vi "PicowattAVS47Monitor.vi"() -> ()   [LabVIEW 2018]
uses:
  Utility/Monitor Communication/PicowattAVS47/PicowattAVS47-Cluster.ctl
  Instrument_Setup.vi
  Global/Global Variables/Data_Display_global.vi
panel:
  in  "?":bool
  out "Picowatt AVS47/TS530 Cluster":T1 {"AVS Excitation" items=["no Exc", "3uV", "10uV", "30uV", "100uV", "300uV", "1mV", "3mV"]}
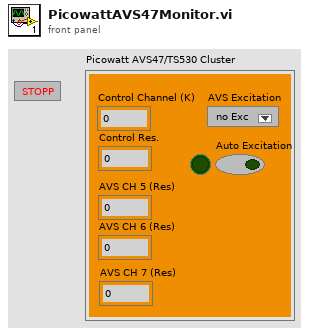
[diagram p1: front panel]
types:
  T1 = typedef "PicowattAVS47-Cluster.ctl" = cluster{"Control Channel (K)":dbl, "AVS CH 5 (Res)":dbl, "AVS CH 6 (Res) ":dbl, "AVS CH 7 (Res) ":dbl, "Control Res.":dbl, "Auto Excitation":bool, "Auto activatet":bool, "AVS Excitation":i16}
  T2 = typedef "AVS-Control-Cluster.ctl" = cluster{"AVS Excitation":i16, "Auto Excitation":bool}
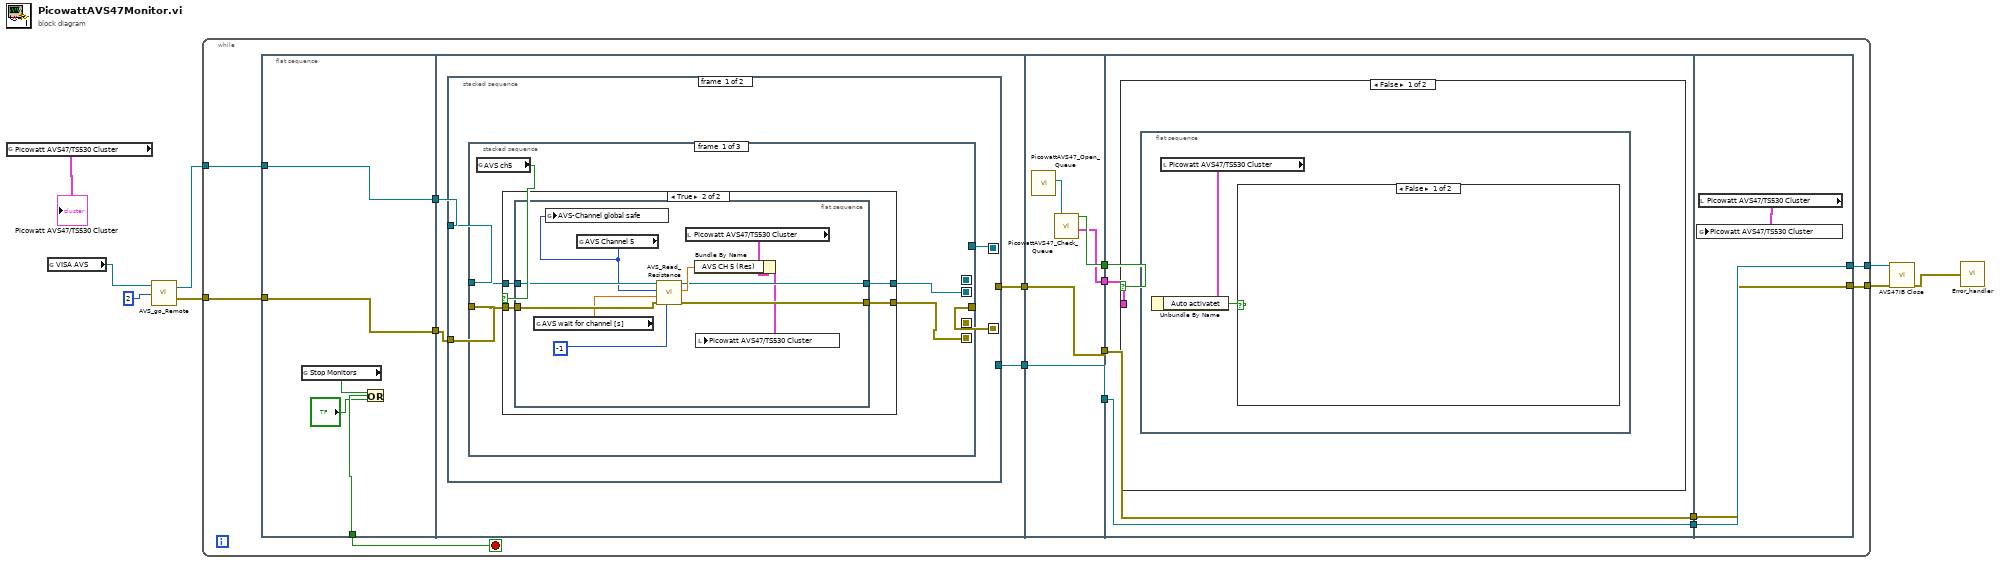
[diagram p0: block diagram]
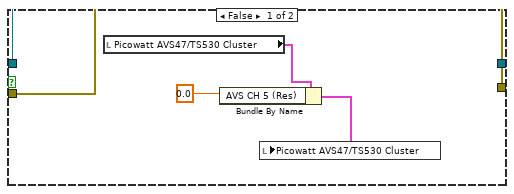
[diagram p2: hidden frame]
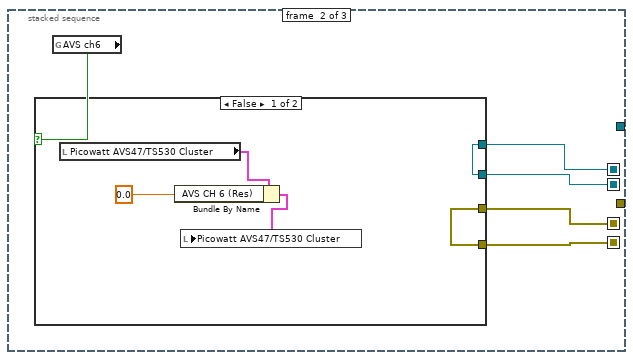
[diagram p3: hidden frame]
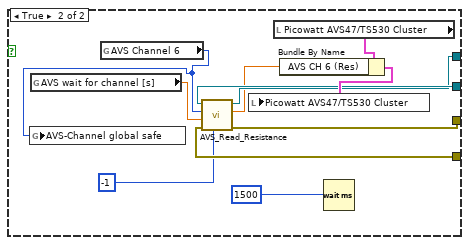
[diagram p4: hidden frame]
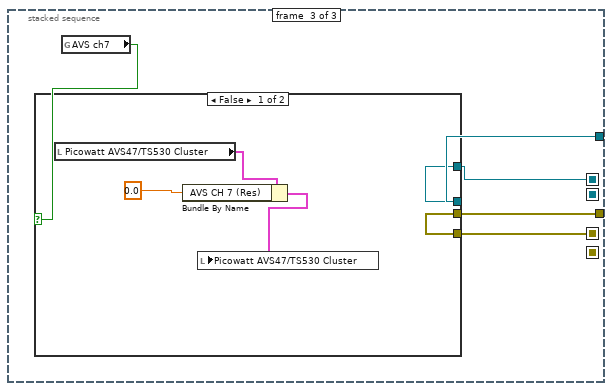
[diagram p5: hidden frame]
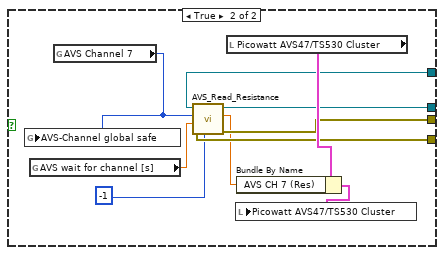
[diagram p6: hidden frame]
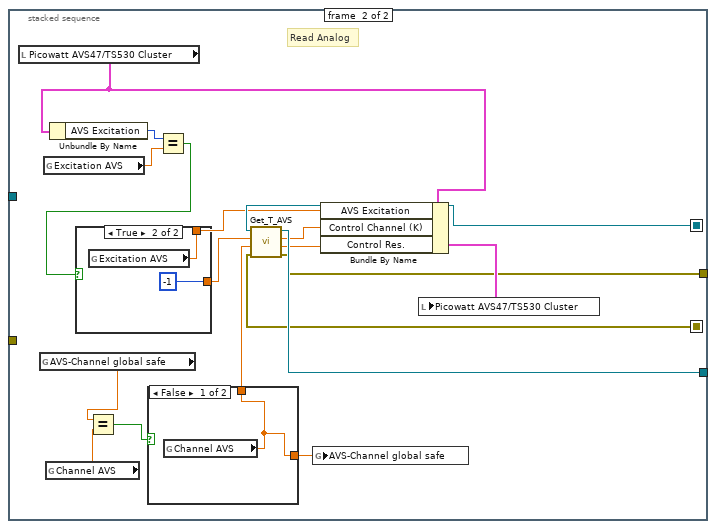
[diagram p7: hidden frame]
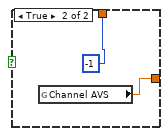
[diagram p8: hidden frame]
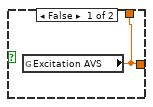
[diagram p9: hidden frame]
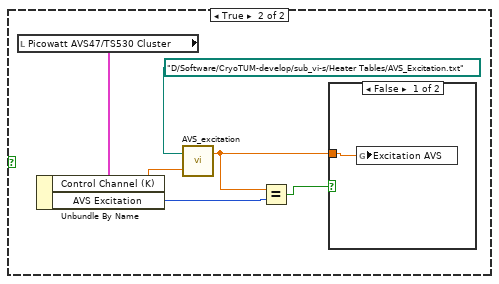
[diagram p10: hidden frame]
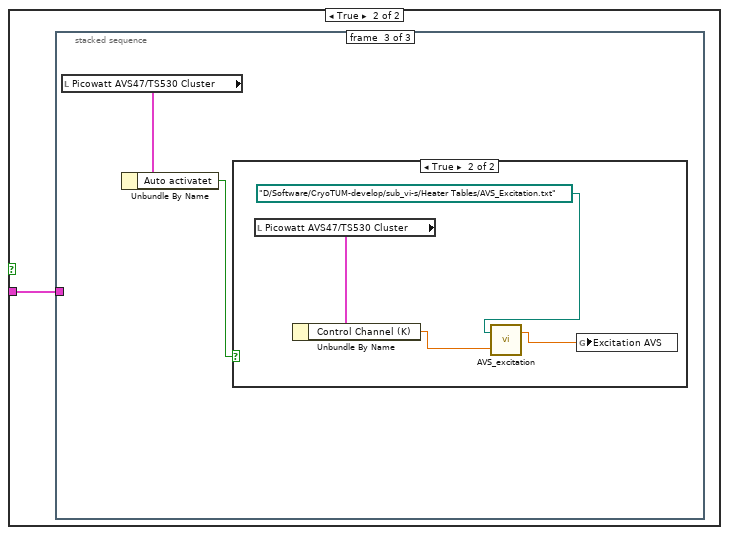
[diagram p12: hidden frame]
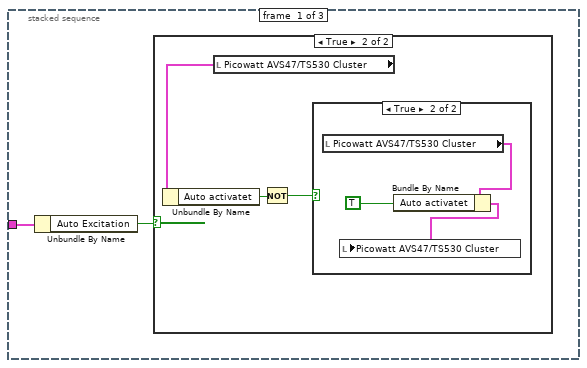
[diagram p13: hidden frame]
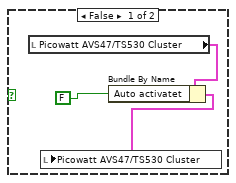
[diagram p15: hidden frame]
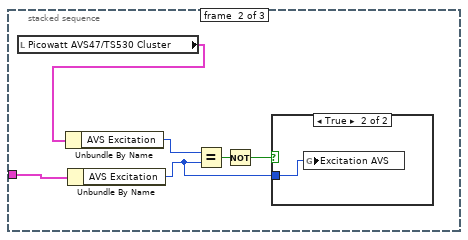
[diagram p16: hidden frame]
diagram:
  n1 = global read "Data_Display_global.vi" "Picowatt AVS47/TS530 Cluster"() -> (→"Picowatt AVS47/TS530 Cluster":T1)
  n2 = global read "Instrument_Setup.vi" "VISA AVS"() -> (w7:refnum<visa-resource-name>)
  n3 = call "AVS_go_Remote.vi"("Timeout (sec)"=i16 2, "VISA-AVS"=w7) -> ("error out"=w8:errorcluster, "dup VISA session"=w6:refnum<visa-resource-name>)  [unwired: 1 in]
  n4 = while {
    tunnel: w8 -> [w18]
    tunnel: w6 -> [w17]
    tunnel: [w10] -> w3
    tunnel: [w9] -> w2
    stop <- w23 stop-if-true
    n5 = flat-sequence {
      tunnel: [w28] -> w23
      tunnel: [w24] -> w22
      tunnel: [w25] -> w19
      tunnel: w18 -> [w25]
      tunnel: w17 -> [w24]
      tunnel: w22 -> [w32]
      tunnel: w19 -> [w31]
      tunnel: [w30] -> w16
      tunnel: [w29] -> w15
      tunnel: [w129] -> w21
      tunnel: [w128] -> w20
      tunnel: w16 -> [w126]
      tunnel: w15 -> [w127]
      tunnel: [w127] -> w14
      tunnel: [w126] -> w13
      tunnel: w21 -> [w134]
      tunnel: w20 -> [w133]
      tunnel: w14 -> [w131]
      tunnel: w13 -> [w132]
      tunnel: [w132] -> w12
      tunnel: [w131] -> w11
      tunnel: w12 -> [w170]
      tunnel: w11 -> [w169]
      tunnel: [w170] -> w10
      tunnel: [w169] -> w9
      frame #0 {
        n6 = global read "Data_Display_global.vi" "Stop Monitors"() -> (w26:bool)
        n7 = Or(x=w26, y="?") -> (x .or. y?=w28:bool)
      }
      frame #1 {
        n8 = stacked-sequence {
          seq-local: [w34 _] -> [_ w118]
          seq-local: [w33 _] -> [_ w116]
          tunnel: w32 -> [w35 _]
          tunnel: w31 -> [w36 _]
          tunnel: [_ w117] -> w30
          tunnel: [_ w115] -> w29
          frame #0 {
            n9 = stacked-sequence {
              seq-local: [w40 _ _] -> [_ w64 _]
              seq-local: [_ w63 _] -> [_ _ w85]
              seq-local: [w37 _ _] -> [_ w62 _]
              seq-local: [_ w61 _] -> [_ _ w83]
              tunnel: w36 -> [w39 _ _]
              tunnel: [_ _ w84] -> w33
              tunnel: w35 -> [w38 _ _]
              tunnel: [_ _ w82] -> w34
              frame #0 {
                n10 = global read "Instrument_Setup.vi" "AVS ch5"() -> (w41:bool)
                n11 = case shown="True" w41 {
                  tunnel: [w46 w50] -> w40
                  tunnel: w39 -> [w46 w49]
                  tunnel: w38 -> [w45 w48]
                  tunnel: [w45 w47] -> w37
                  frame False {
                    n12 = local read "Picowatt AVS47/TS530 Cluster"() -> (w44:T1)
                    n13 = Bundle By Name(cluster=w44, "AVS CH 5 (Res)"=0.0) -> (w42:T1)
                    n14 = local write "Picowatt AVS47/TS530 Cluster"(w42) -> ()
                  }
                  frame True {
                    n15 = flat-sequence {
                      tunnel: w49 -> [w58]
                      tunnel: w48 -> [w57]
                      tunnel: [w59] -> w50
                      tunnel: [w54] -> w47
                      frame #0 {
                        n16 = global read "Instrument_Setup.vi" "AVS wait for channel [s]"() -> (w56:dbl)
                        n17 = global read "Instrument_Setup.vi" "AVS Channel 5"() -> (w52:enum16{"1", "2", "3", "4", "5", "6", "7"})
                        n18 = global write "Data_Display_global.vi" "AVS-Channel global safe"(w52) -> ()
                        n19 = call "AVS_Read_Resistance.vi"("AVS-Excitation"=i8 -1, "error in (no error)"=w58, "Wait for channel (s)"=w56, "AVS Channel"=w52, "AVS-VISA"=w57) -> ("error out"=w59:errorcluster, "AVS Resistance reading"=w55:dbl, "dup AVS-VISA"=w54:refnum<visa-resource-name>)  [unwired: 2 in]
                        n20 = local read "Picowatt AVS47/TS530 Cluster"() -> (w60:T1)
                        n21 = Bundle By Name(cluster=w60, "AVS CH 5 (Res)"=w55) -> (w51:T1)
                        n22 = local write "Picowatt AVS47/TS530 Cluster"(w51) -> ()
                      }
                    }
                  }
                }
              }
              frame #1 {
                n23 = global read "Instrument_Setup.vi" "AVS ch6"() -> (w65:bool)
                n24 = case shown="False" w65 {
                  tunnel: w64 -> [w70 w79]
                  tunnel: [w70 w78] -> w63
                  tunnel: w62 -> [w69 w77]
                  tunnel: [w69 w76] -> w61
                  frame False {
                    n25 = local read "Picowatt AVS47/TS530 Cluster"() -> (w68:T1)
                    n26 = Bundle By Name(cluster=w68, "AVS CH 6 (Res)"=0.0) -> (w66:T1)
                    n27 = local write "Picowatt AVS47/TS530 Cluster"(w66) -> ()
                  }
                  frame True {
                    n28 = global read "Instrument_Setup.vi" "AVS wait for channel [s]"() -> (w75:dbl)
                    n29 = global read "Instrument_Setup.vi" "AVS Channel 6"() -> (w72:enum16{"1", "2", "3", "4", "5", "6", "7"})
                    n30 = global write "Data_Display_global.vi" "AVS-Channel global safe"(w72) -> ()
                    n31 = call "AVS_Read_Resistance.vi"("AVS-Excitation"=i8 -1, "error in (no error)"=w79, "Wait for channel (s)"=w75, "AVS Channel"=w72, "AVS-VISA"=w77) -> ("error out"=w78:errorcluster, "AVS Resistance reading"=w74:dbl, "dup AVS-VISA"=w76:refnum<visa-resource-name>)  [unwired: 2 in]
                    n32 = local read "Picowatt AVS47/TS530 Cluster"() -> (w81:T1)
                    n33 = Bundle By Name(cluster=w81, "AVS CH 6 (Res)"=w74) -> (w80:T1)
                    n34 = local write "Picowatt AVS47/TS530 Cluster"(w80) -> ()
                    n35 = Wait (ms)(milliseconds to wait=1500) -> ()  [unwired: 1 out]
                  }
                }
              }
              frame #2 {
                n36 = global read "Instrument_Setup.vi" "AVS ch7"() -> (w86:bool)
                n37 = case shown="False" w86 {
                  tunnel: w85 -> [w91 w100]
                  tunnel: [w91 w99] -> w84
                  tunnel: w83 -> [w90 w98]
                  tunnel: [w90 w97] -> w82
                  frame False {
                    n38 = local read "Picowatt AVS47/TS530 Cluster"() -> (w89:T1)
                    n39 = Bundle By Name(cluster=w89, "AVS CH 7 (Res)"=0.0) -> (w87:T1)
                    n40 = local write "Picowatt AVS47/TS530 Cluster"(w87) -> ()
                  }
                  frame True {
                    n41 = global read "Instrument_Setup.vi" "AVS wait for channel [s]"() -> (w96:dbl)
                    n42 = global read "Instrument_Setup.vi" "AVS Channel 7"() -> (w93:enum16{"1", "2", "3", "4", "5", "6", "7"})
                    n43 = global write "Data_Display_global.vi" "AVS-Channel global safe"(w93) -> ()
                    n44 = call "AVS_Read_Resistance.vi"("AVS-Excitation"=i8 -1, "error in (no error)"=w100, "Wait for channel (s)"=w96, "AVS Channel"=w93, "AVS-VISA"=w98) -> ("error out"=w99:errorcluster, "AVS Resistance reading"=w95:dbl, "dup AVS-VISA"=w97:refnum<visa-resource-name>)  [unwired: 2 in]
                    n45 = local read "Picowatt AVS47/TS530 Cluster"() -> (w101:T1)
                    n46 = Bundle By Name(cluster=w101, "AVS CH 7 (Res)"=w95) -> (w92:T1)
                    n47 = local write "Picowatt AVS47/TS530 Cluster"(w92) -> ()
                  }
                }
              }
            }
          }
          frame #1 {
            # "Read Analog"
            n48 = local read "Picowatt AVS47/TS530 Cluster"() -> (w102:T1)
            n49 = global read "Data_Display_global.vi" "AVS-Channel global safe"() -> (w108:dbl)
            n50 = global read "Instrument_Setup.vi" "Excitation AVS"() -> (w111:dbl)
            n51 = global read "Instrument_Setup.vi" "Channel AVS"() -> (w107:dbl)
            n52 = Unbundle By Name(w102) -> ("AVS Excitation"=w112:i16)
            n53 = Equal?(x=w108, y=w107) -> (x = y?=w106:bool)
            n54 = case shown="False" w106 {
              tunnel: [w120 -1] -> w105
              tunnel: [w120 w121] -> w104
              frame False {
                n55 = global read "Instrument_Setup.vi" "Channel AVS"() -> (w120:dbl)
              }
              frame True {
                n56 = global read "Instrument_Setup.vi" "Channel AVS"() -> (w121:dbl)
              }
            }
            n57 = Equal?(x=w112, y=w111) -> (x = y?=w110:bool)
            n58 = case shown="True" w110 {
              tunnel: [w123 -1] -> w109
              tunnel: [w123 w124] -> w103
              frame False {
                n59 = global read "Instrument_Setup.vi" "Excitation AVS"() -> (w123:dbl)
              }
              frame True {
                n60 = global read "Instrument_Setup.vi" "Excitation AVS"() -> (w124:dbl)
              }
            }
            n61 = call "Get_T_AVS.vi"("error in (no error)"=w116, "AVS-Channel"=w105, "AVS-Excitation"=w109, "AVS-VISA"=w118) -> ("error out"=w115:errorcluster, "Resistance reading"=w113:dbl, "T (K)"=w114:dbl, "dup AVS-VISA"=w117:refnum<visa-resource-name>)
            n62 = global write "Data_Display_global.vi" "AVS-Channel global safe"(w104) -> ()
            n63 = Bundle By Name(cluster=w102, "AVS Excitation"=w103, "Control Channel (K)"=w114, "Control Res."=w113) -> (w119:T1)
            n64 = local write "Picowatt AVS47/TS530 Cluster"(w119) -> ()
          }
        }
      }
      frame #2 {
        n65 = call "PicowattAVS47_Open_Queue.vi"() -> ("queue out"=w130:refnum<queue>)  [unwired: 10 in, 1 out]
        n66 = call "PicowattAVS47_Check_Queue.vi"("queue"=w130) -> ("AVS47 Control Cluster"=w128:T2, "New Entries ?"=w129:bool)  [unwired: 7 in, 1 out]
      }
      frame #3 {
        n67 = case shown="False" w134 {
          tunnel: w133 -> [_ w144]
          frame False {
            n68 = flat-sequence {
              frame #0 {
                n69 = local read "Picowatt AVS47/TS530 Cluster"() -> (w135:T1)
                n70 = Unbundle By Name(w135) -> ("Auto activatet"=w136:bool)
                n71 = case shown="False" w136 {
                  frame False {
                  }
                  frame True {
                    n72 = local read "Picowatt AVS47/TS530 Cluster"() -> (w141:T1)
                    n73 = Unbundle By Name(w141) -> ("Control Channel (K)"=w140:dbl, "AVS Excitation"=w139:i16)
                    n74 = call "AVS_excitation.vi"("AVS-Temperatur"=w140, "Pfad"=path "D:/Software/CryoTUM-develop/sub_vi-s/Heater Tables/AVS_Excitation.txt") -> ("Excitation AVS"=w137:dbl)  [unwired: 1 in]
                    n75 = Equal?(x=w137, y=w139) -> (x = y?=w138:bool)
                    n76 = case shown="False" w138 {
                      tunnel: w137 -> [w143 _]
                      frame False {
                        n77 = global write "Instrument_Setup.vi" "Excitation AVS"(w143) -> ()
                      }
                      frame True {
                      }
                    }
                  }
                }
              }
            }
          }
          frame True {
            n78 = stacked-sequence {
              tunnel: w144 -> [w146 w161 _]
              frame #0 {
                n79 = Unbundle By Name(w146) -> ("Auto Excitation"=w145:bool)
                n80 = case shown="True" w145 {
                  frame False {
                  }
                  frame True {
                    n81 = local read "Picowatt AVS47/TS530 Cluster"() -> (w149:T1)
                    n82 = Unbundle By Name(w149) -> ("Auto activatet"=w147:bool)
                    n83 = Not(x=w147) -> (.not. x?=w148:bool)
                    n84 = case shown="True" w148 {
                      frame False {
                        n85 = local read "Picowatt AVS47/TS530 Cluster"() -> (w152:T1)
                        n86 = Bundle By Name(cluster=w152, "Auto activatet"=FALSE) -> (w151:T1)
                        n87 = local write "Picowatt AVS47/TS530 Cluster"(w151) -> ()
                      }
                      frame True {
                        n88 = local read "Picowatt AVS47/TS530 Cluster"() -> (w155:T1)
                        n89 = Bundle By Name(cluster=w155, "Auto activatet"=TRUE) -> (w154:T1)
                        n90 = local write "Picowatt AVS47/TS530 Cluster"(w154) -> ()
                      }
                    }
                  }
                }
              }
              frame #1 {
                n91 = local read "Picowatt AVS47/TS530 Cluster"() -> (w160:T1)
                n92 = Unbundle By Name(w160) -> ("AVS Excitation"=w159:i16)
                n93 = Unbundle By Name(w161) -> ("AVS Excitation"=w156:i16)
                n94 = Equal?(x=w159, y=w156) -> (x = y?=w158:bool)
                n95 = Not(x=w158) -> (.not. x?=w157:bool)
                n96 = case shown="True" w157 {
                  tunnel: w156 -> [_ w162]
                  frame False {
                  }
                  frame True {
                    n97 = global write "Instrument_Setup.vi" "Excitation AVS"(w162) -> ()
                  }
                }
              }
              frame #2 {
                n98 = local read "Picowatt AVS47/TS530 Cluster"() -> (w164:T1)
                n99 = Unbundle By Name(w164) -> ("Auto activatet"=w163:bool)
                n100 = case shown="True" w163 {
                  frame False {
                  }
                  frame True {
                    n101 = local read "Picowatt AVS47/TS530 Cluster"() -> (w167:T1)
                    n102 = Unbundle By Name(w167) -> ("Control Channel (K)"=w166:dbl)
                    n103 = call "AVS_excitation.vi"("AVS-Temperatur"=w166, "Pfad"=path "D:/Software/CryoTUM-develop/sub_vi-s/Heater Tables/AVS_Excitation.txt") -> ("Excitation AVS"=w168:dbl)  [unwired: 1 in]
                    n104 = global write "Instrument_Setup.vi" "Excitation AVS"(w168) -> ()
                  }
                }
              }
            }
          }
        }
      }
      frame #4 {
        n105 = local read "Picowatt AVS47/TS530 Cluster"() -> (w171:T1)
        n106 = global write "Data_Display_global.vi" "Picowatt AVS47/TS530 Cluster"(w171) -> ()
      }
    }
  }
  n107 = call "AVS47IB Close.vi"("VISA session"=w3, "error in (no error)"=w2) -> ("error out"=w4:errorcluster)  [unwired: 13 in]
  n108 = call "Error_handler.vi"("error constant"=w4) -> ()
